vi "sync and trig.vi"(8 "error in (no error)":errorcluster, 11 "pulse_gen_and_detect_p2p in":refnum<class "pulse_gen_and_detect_p2p.lvclass">) -> (0 "error out":errorcluster, 3 "pulse_gen_and_detect_p2p out":refnum<class "pulse_gen_and_detect_p2p.lvclass">)   [LabVIEW 2021, in "pulse_gen_and_detect_p2p.lvclass"]
uses:
  pulse_gen_and_detect_p2p.lvclass
  pulse_gen_and_detect_p2p.lvclass/pulse_gen_and_detect_p2p.ctl
  <vilib>/rvi/interface/nirviReadWriteControl/nirviReadWriteControl.xnode
  NiFpgaLv.dll
  <vilib>/Utility/error.llb/Error Cluster From Error Code.vi
  <vilib>/rvi/interface/Simulation/niFpgaSimulationCallBeginRW.vi
  <vilib>/rvi/errors/niLvFpgaAdjustHostInterfaceError.vi
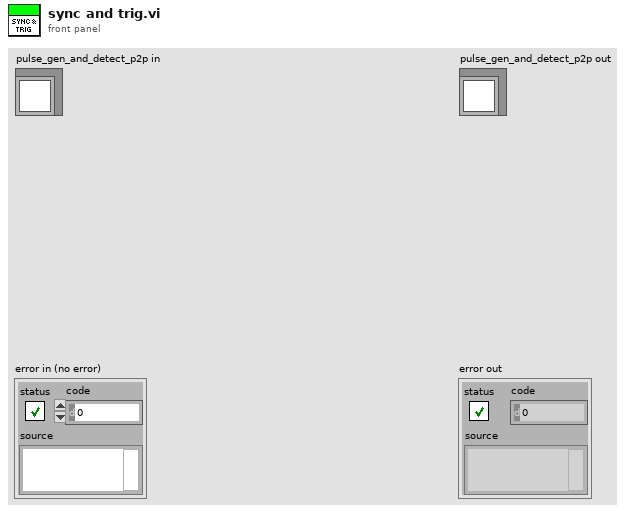
[diagram p1: front panel]
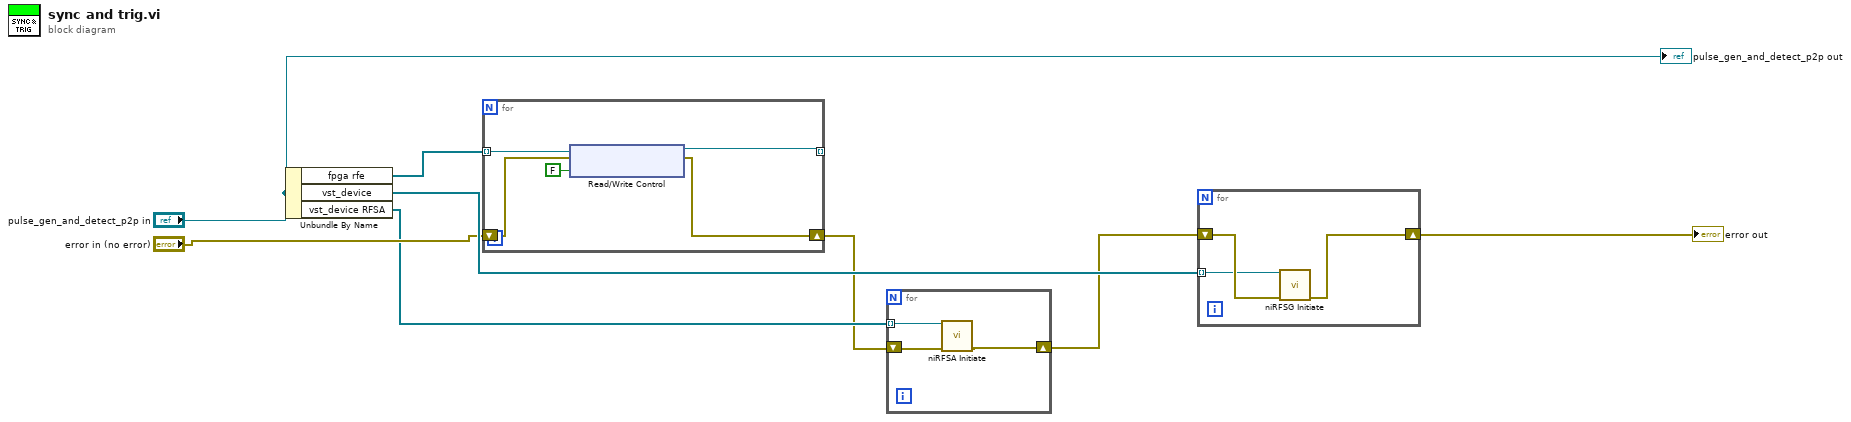
[diagram p0: block diagram]
diagram:
  n1 = Unbundle By Name("pulse_gen_and_detect_p2p in") -> ("fpga rfe"=w8:refnum<k20>[], "vst_device"=w7:refnum<k15>[], "vst_device RFSA"=w3:refnum<k15>[])
  n2 = for {
    tunnel: w8 -> [w13] mode=indexing
    tunnel: [w12] -> _ mode=indexing
    shift-right: [w9] -> w2
    shift-left: "error in (no error)" -> [w11]
    n3 = xnode "Read/Write Control"("FPGA VI Reference In"=w13, "error in"=w11, "reset system clock"=FALSE) -> ("FPGA VI Reference Out"=w12:refnum<k20>, "error out"=w9:errorcluster)
  }
  n4 = for {
    tunnel: w3 -> [w16] mode=indexing
    shift-right: [w14] -> w1
    shift-left: w2 -> [w15]
    n5 = call <instrlib>:"niRFSA Initiate.vi"("instrument handle"=w16, "error in"=w15) -> ("error out"=w14:errorcluster)  [unwired: 12 in, 1 out]
  }
  n6 = for {
    shift-right: [w18] -> w4
    shift-left: w1 -> [w19]
    tunnel: w7 -> [w17] mode=indexing
    n7 = call <instrlib>:"niRFSG Initiate.vi"("instrument handle"=w17, "error in"=w19) -> ("error out"=w18:errorcluster)  [unwired: 12 in, 1 out]
  }
  "error out" <- w4
  "pulse_gen_and_detect_p2p out" <- "pulse_gen_and_detect_p2p in"
